vi "Load Flattened Image from Tiff.vi"(0 "path to TIFF file":path=path "/HD1/Users/herbertlooser/Desktop/LadungssprŸher.tif", 1 "error in (no error)":errorcluster) -> (5 "image data":T1, 7 "error out":errorcluster)   [LabVIEW 2012, in "TIFF File Reader.lvlib"]
uses:
  TIFF File Reader.lvlib
  <vilib>/picture/picture.llb/imagedata.ctl
  Globals.vi
panel:
  in  "Tab Control":T2(tab)
  out "Grayscale":picture
  out "Gray16/32":sgl[][](array[numeric])
  out "N_Bits":u64
  out "Gray8":u8[][](array[numeric])
  out "GrayWithLUT":picture
  out "Gray8 LUT":u8[][](array[numeric])
  out "RGB":picture
  out "N_RGB_Bits":u64
  out "R16/32":sgl[][](array[numeric])
  out "G16/32":sgl[][](array[numeric])
  out "B16/32":sgl[][](array[numeric])
  out "RGB8":u32[][](array[numeric])
  out "PhotoM":T3(ring)=enum."BlackIsZero"
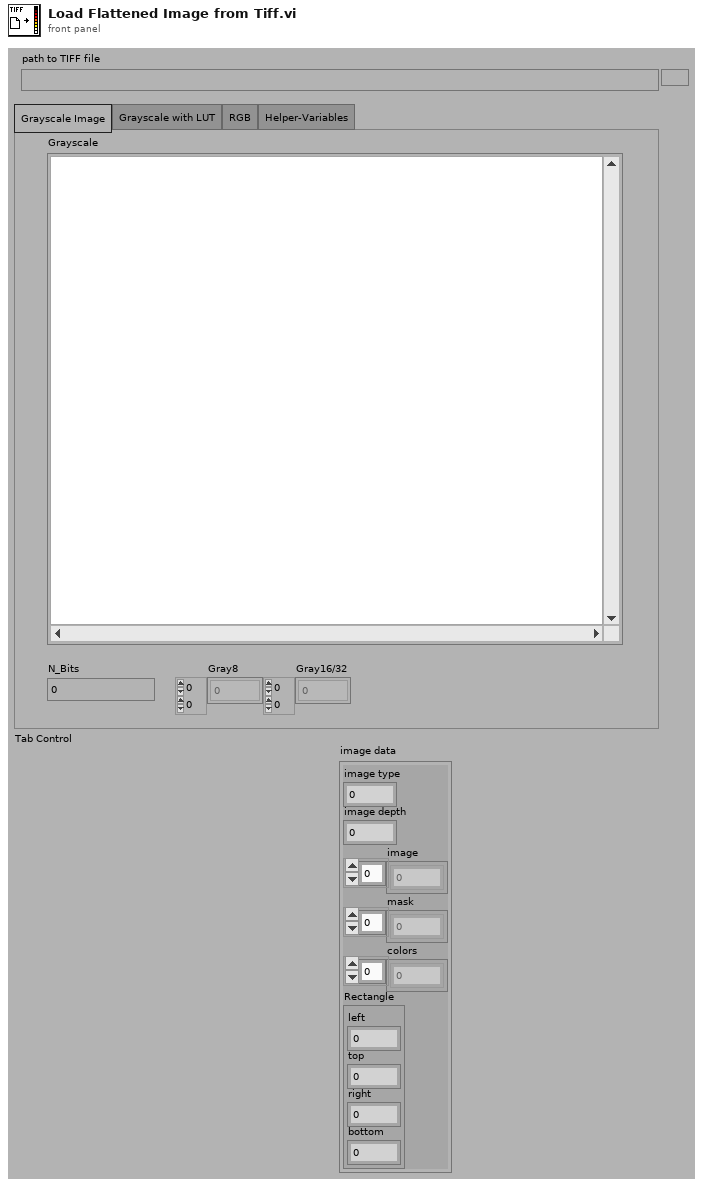
[diagram p1: front panel]
types:
  T1 = typedef "imagedata.ctl" = cluster{"image type":i32, "image depth":i32, "image":u8[], "mask":u8[], "colors":u32[], "Rectangle":cluster{"left":i16, "top":i16, "right":i16, "bottom":i16}}
  T2 = enum32{"Grayscale Image", "Grayscale with LUT", "RGB", "Helper-Variables"}
  T3 = enum16{"WhiteIsZero", "BlackIsZero", "RGB", "RGBPalette", "TranspMask", "CMYK", "YCbCr", "Null", "CIELab"}
  T4 = enum16{"open", "open or create", "create or replace", "create"}
  T5 = enum32{"existing file", "new file", "new or existing file", "existing dir", "new dir", "new or existing dir", "existing file (use LLBs)", "new file (use LLBs)", "new or existing file (use LLBs)", "new or existing file or directory (use LLBs)", "existing dir (use LLBs)", "new dir (use LLBs)", "new or existing dir (use LLBs)", "existing file or dir", "new file or dir", "new or existing file or dir", "existing file or dir (use LLBs)", "new file or dir (use LLBs)"}
  T6 = typedef "TIFF File Reader.lvlib/IFD Entry.ctl" = cluster{"Tag":u16, "Type":T7, "Count":u32, "Val/Offs":u32, "Is Val/Offs(T)":bool}
  T7 = typedef "TIFF File Reader.lvlib/FieldTypes.ctl" = enum16{"NULL", "U8", "ASCII7", "U16", "U32", "RATIONAL", "SByte(I8)", "Undef(8Bit)", "I16", "I32", "SRat(4B:4B)", "SGL(4Byte)", "DBL(8Byte)"}
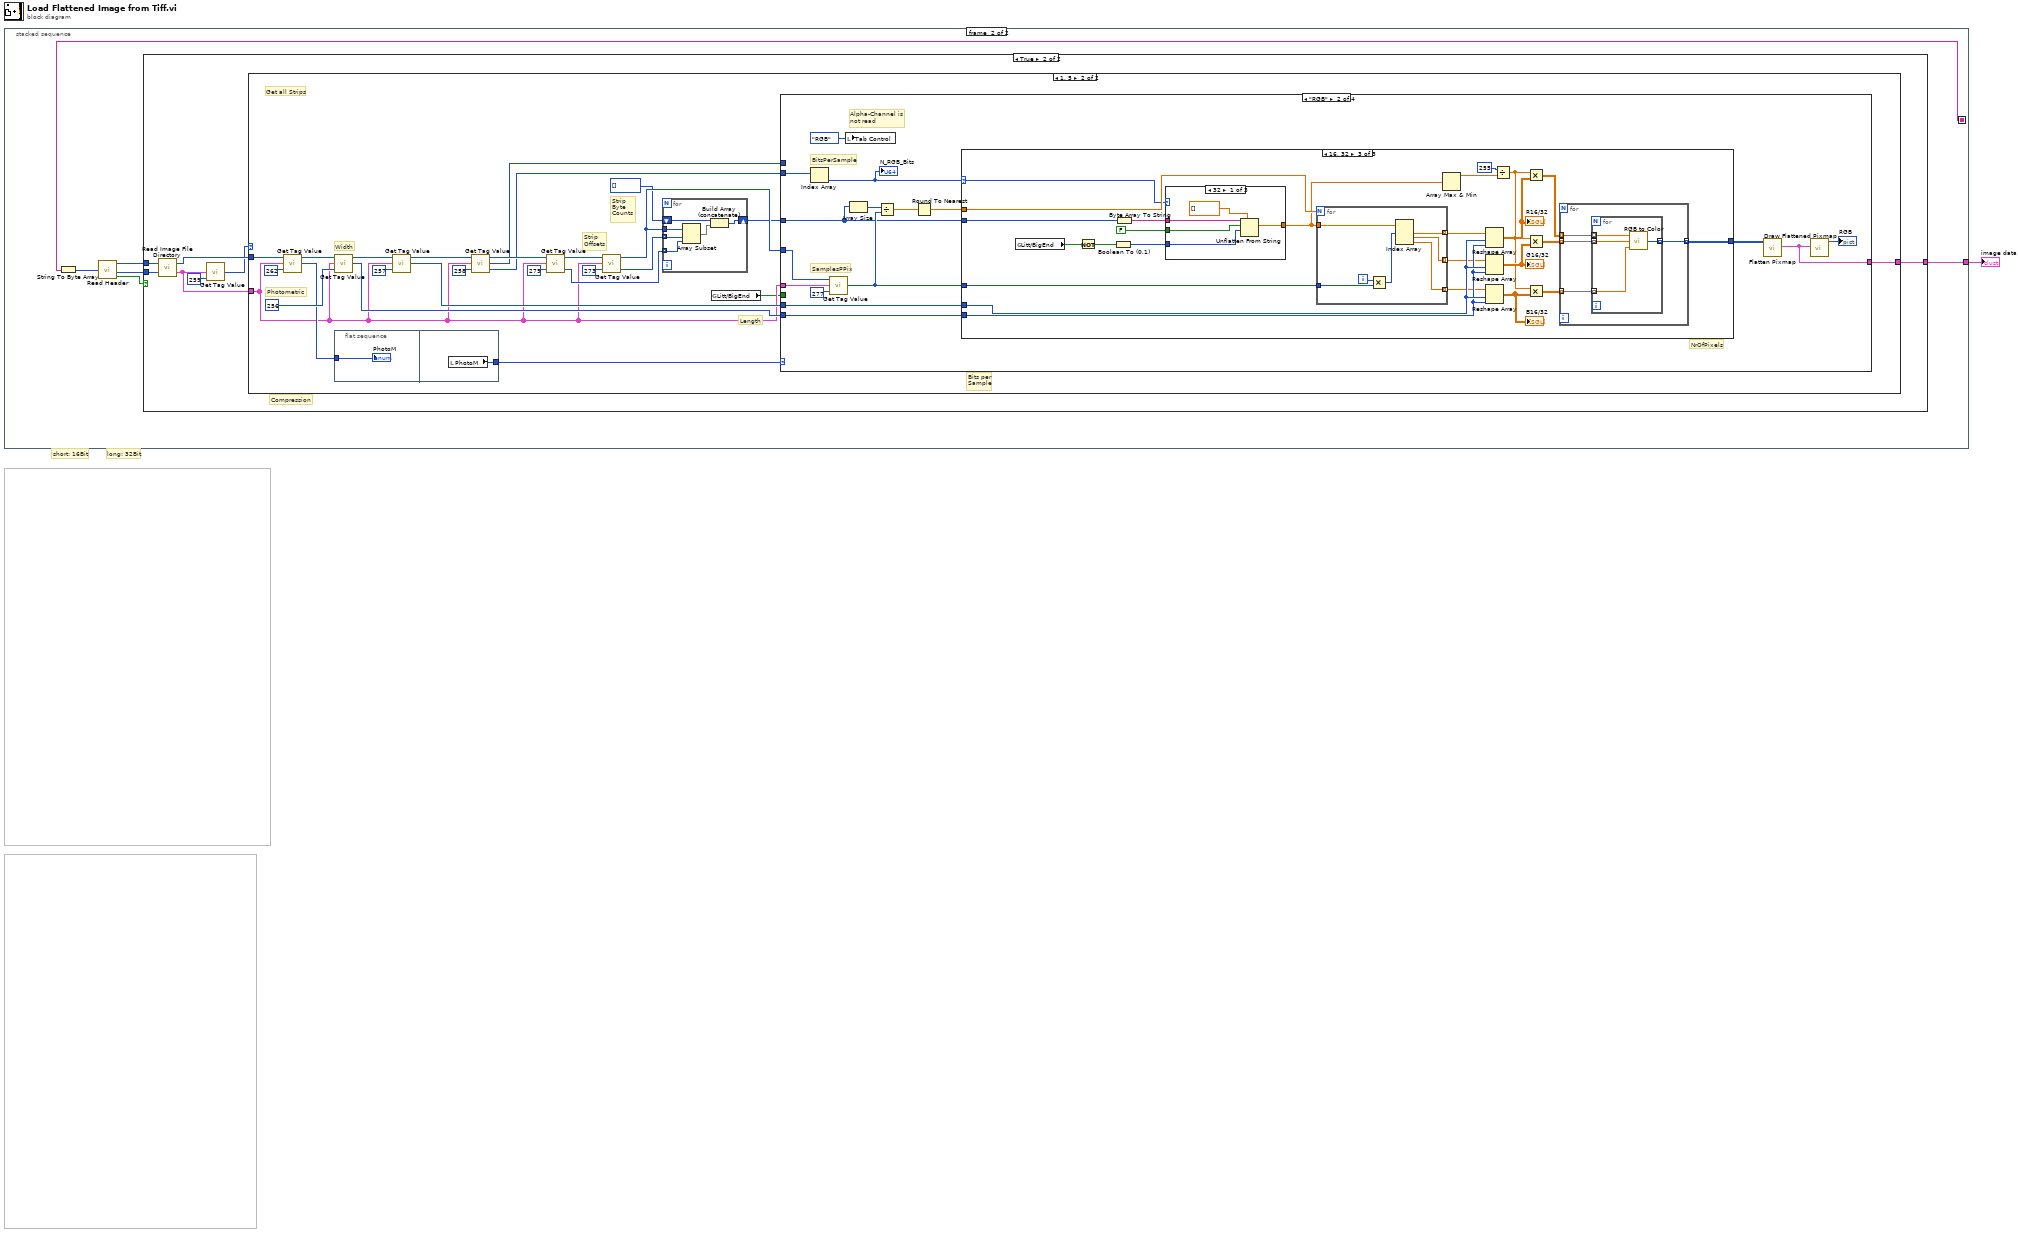
[diagram p0: block diagram]
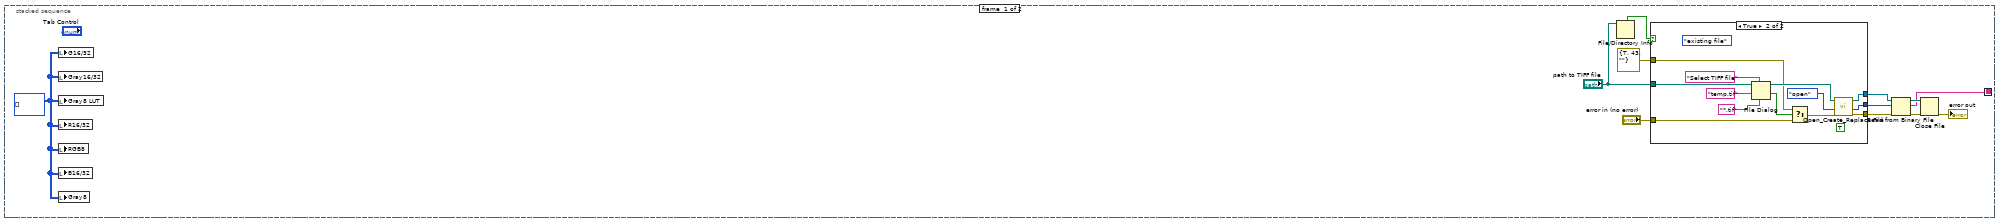
[diagram p2: hidden frame]
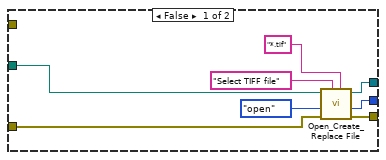
[diagram p3: hidden frame]
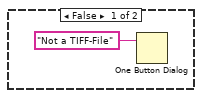
[diagram p4: hidden frame]
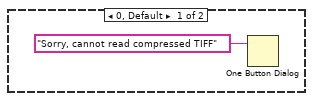
[diagram p5: hidden frame]
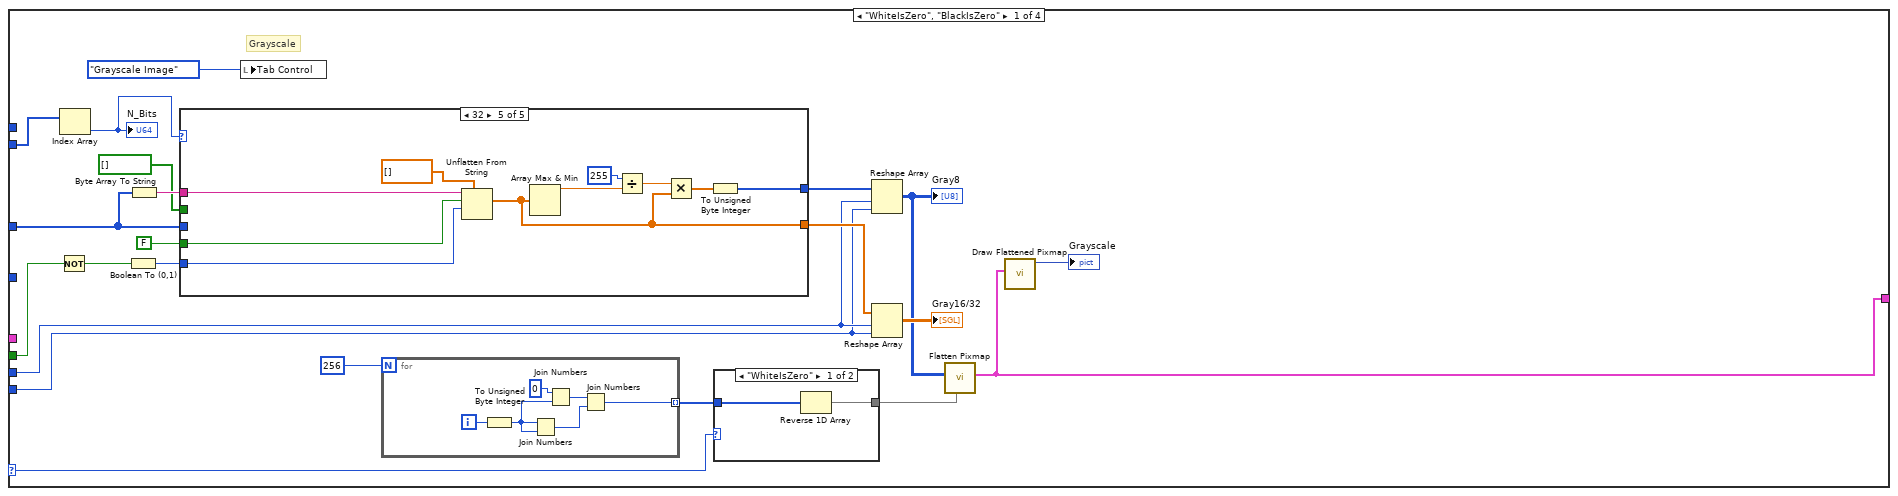
[diagram p6: hidden frame]
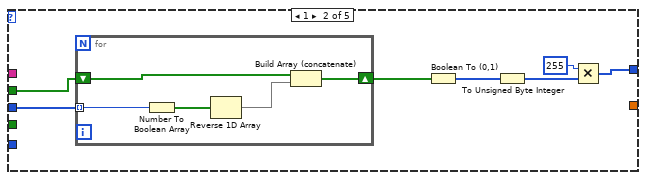
[diagram p9: hidden frame]
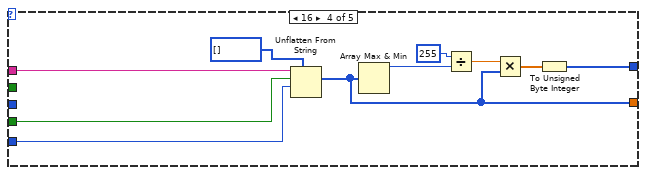
[diagram p11: hidden frame]
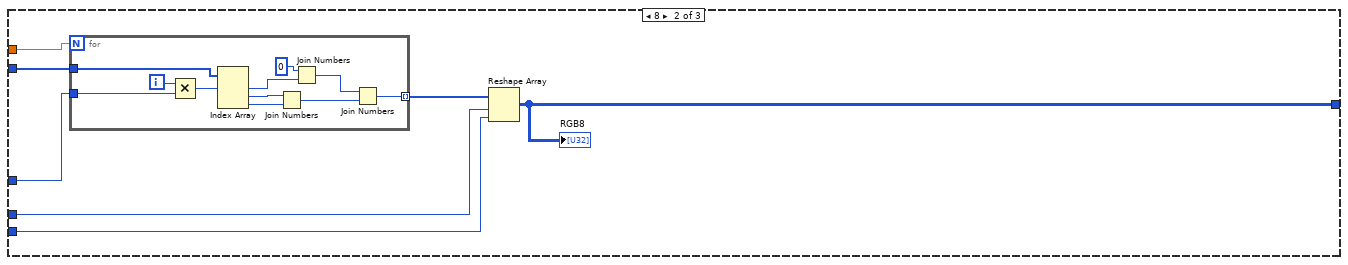
[diagram p13: hidden frame]
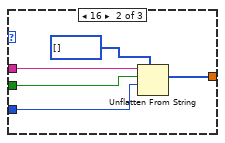
[diagram p14: hidden frame]
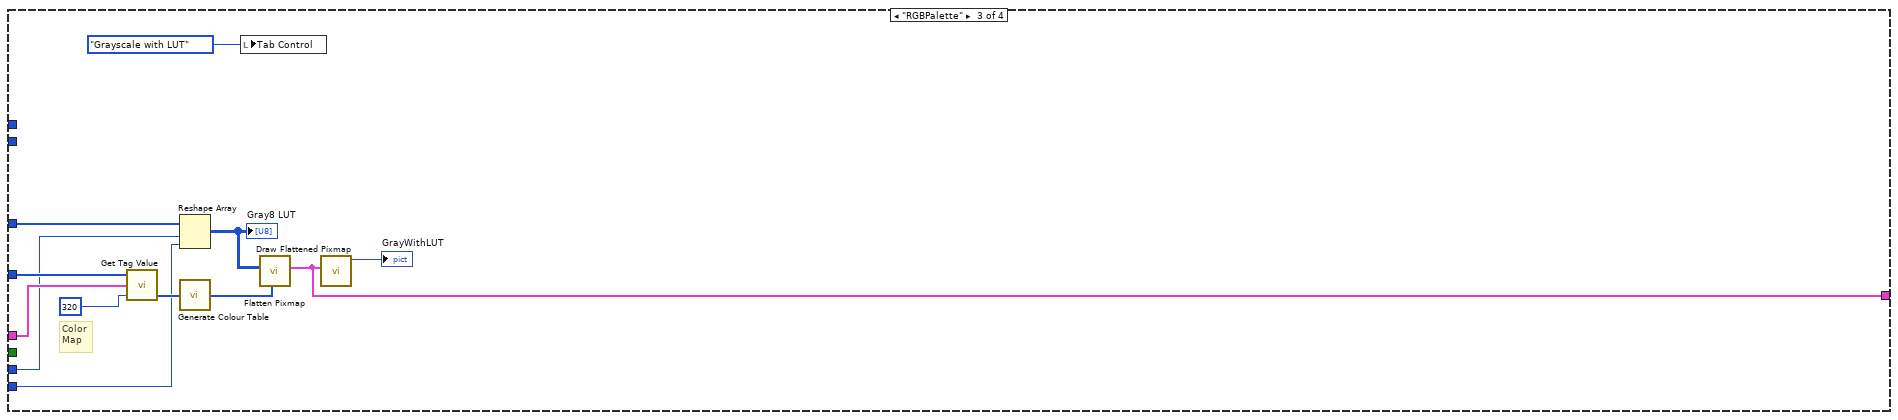
[diagram p16: hidden frame]
diagram:
  # "long: 32Bit"
  # "short: 16Bit"
  n1 = stacked-sequence {
    seq-local: [w3 _] -> [_ w39]
    tunnel: [_ w35] -> w1
    frame #0 {
      w2 = u32[][] [] ("RGB8")
      n2 = local write "G16/32"(w2) -> ()
      n3 = local write "Gray16/32"(w2) -> ()
      n4 = local write "Gray8 LUT"(w2) -> ()
      n5 = local write "R16/32"(w2) -> ()
      n6 = local write "RGB8"(w2) -> ()
      n7 = local write "B16/32"(w2) -> ()
      n8 = local write "Gray8"(w2) -> ()
      n9 = File/Directory Info(path="path to TIFF file") -> (directory=w7:bool)  [unwired: 1 in, 6 out]
      n10 = case shown="True" w7 {
        tunnel: [w18 w27] -> w13
        tunnel: [w17 w29] -> w12
        tunnel: [w16 w28] -> w9
        tunnel: "error in (no error)" -> [w15 w25]
        tunnel: "path to TIFF file" -> [w14 w22]
        tunnel: errorcluster {"status"=TRUE, "code"=43, "source"=""} ("error in (no error)") -> [_ w23]
        frame False {
          n11 = call <vilib>:"Open_Create_Replace File.vi"("pattern"="*.tif", "prompt"="Select TIFF file", "error in (no error)"=w15, "function (open:0)"=T4."open", "file path"=w14) -> ("error out"=w16:errorcluster, "file size (bytes)"=w18:i32, "refnum"=w17:refnum<file>)  [unwired: 2 in, 2 out]
        }
        frame True {
          (unwired) T5."existing file" ("select mode (2)")
          (unwired) TRUE ("advisory dialog? (display:T)")
          n12 = File Dialog(6:"*.tif" ("pattern"), 7:"Select TIFF file" ("prompt"), 9:"temp.tif" ("default name"), 11:w22) -> (1:w26:bool, 3:w31:path)  [unwired: 1 in, 4 out]
          n13 = Select(t=w23, s=w26, f=w25) -> (s? t:f=w24:errorcluster)
          n14 = call <vilib>:"Open_Create_Replace File.vi"("error in (no error)"=w24, "function (open:0)"=T4."open", "file path"=w31) -> ("error out"=w28:errorcluster, "file size (bytes)"=w27:i32, "refnum"=w29:refnum<file>)  [unwired: 3 in, 3 out]
        }
      }
      n15 = Read from Binary File(8:w9, 10:w13, 11:w12) -> (0:w10:errorcluster, 2:w3:string, 3:w11:refnum<file>)  [unwired: 4 out]
      n16 = Close File(refnum=w11, error in=w10) -> (error out=→"error out":errorcluster)  [unwired: 1 out]
    }
    frame #1 {
      n17 = String To Byte Array(string=w39) -> (unsigned byte array=w40:u8[])
      n18 = call "Read Header.vi"("Image Data in"=w40) -> ("Image Data out"=w38:u8[], "ImFileDirectOffs"=w37:u32, "isTIFF"=w36:bool)  [unwired: 1 out]
      n19 = case shown="True" w36 {
        tunnel: w38 -> [_ w48]
        tunnel: w37 -> [_ w47]
        tunnel: [_ w42] -> w35
        frame False {
          n20 = One Button Dialog(message="Not a TIFF-File") -> ()  [unwired: 2 out]
        }
        frame True {
          # "Compression"
          n21 = call "Read Image File Directory.vi"("Im_File_Dir Offs"=w47, "Image Data in"=w48) -> ("Directory"=w43:T6[], "Image Data out"=w46:u8[])
          n22 = call "Get Tag Value.vi"("Tag Code"=u16 259, "DirEntries"=w43) -> ("Single Value"=w44:u32)  [unwired: 1 in, 2 out]
          n23 = case shown="1, 5" w44 {
            tunnel: w46 -> [_ w70]
            tunnel: w43 -> [_ w52]
            tunnel: [_ w50] -> w42
            frame 0, Default {
              n24 = One Button Dialog(message="Sorry, cannot read compressed TIFF") -> ()  [unwired: 2 out]
            }
            frame 1, 5 {
              # "Get all Strips"
              # "Strip\nOffsets"
              # "Strip\nByte\nCounts"
              # "Bits per\nSample"
              # "Photometric"
              # "Length"
              # "Width"
              n25 = call "Get Tag Value.vi"("Tag Code"=u16 262, "DirEntries"=w52, "Image Data in"=w70) -> ("Single Value"=w59:u32, "Image Data out"=w69:u8[])  [unwired: 1 out]
              n26 = call "Get Tag Value.vi"("Tag Code"=u16 256, "DirEntries"=w52, "Image Data in"=w69) -> ("Single Value"=w71:u32, "Image Data out"=w75:u8[])  [unwired: 1 out]
              n27 = flat-sequence {
                tunnel: w59 -> [w82]
                tunnel: [w83] -> w58
                frame #0 {
                  "PhotoM" <- w82
                }
                frame #1 {
                  n28 = local read "PhotoM"() -> (w83:T3)
                }
              }
              n29 = call "Get Tag Value.vi"("Tag Code"=u16 257, "DirEntries"=w52, "Image Data in"=w75) -> ("Single Value"=w72:u32, "Image Data out"=w66:u8[])  [unwired: 1 out]
              n30 = call "Get Tag Value.vi"("Tag Code"=u16 258, "DirEntries"=w52, "Image Data in"=w66) -> ("Multiple Values"=w60:u64[], "Single Value"=w61:u32, "Image Data out"=w65:u8[])
              n31 = call "Get Tag Value.vi"("Tag Code"=u16 279, "DirEntries"=w52, "Image Data in"=w65) -> ("Multiple Values"=w55:u64[], "Image Data out"=w64:u8[])  [unwired: 1 out]
              n32 = call "Get Tag Value.vi"("Tag Code"=u16 273, "DirEntries"=w52, "Image Data in"=w64) -> ("Multiple Values"=w56:u64[], "Image Data out"=w57:u8[])  [unwired: 1 out]
              n33 = for {
                tunnel: w57 -> [w81]
                tunnel: w56 -> [w80] mode=indexing
                tunnel: w55 -> [w79] mode=indexing
                shift-right: [w78] -> w53
                shift-left: u8[] [] -> [w76]
                n34 = Array Subset(array=w81, index=w80, length=w79) -> (w77:u8[])
                n35 = Build Array (concatenate)(w76, w77) -> (w78:u8[])
              }
              n36 = global read "Globals.vi" "Litt/BigEnd"() -> (w51:bool)
              n37 = case shown="\"RGB\"" w58 {
                selector: w58 -> [w94 _ _ _]
                tunnel: w72 -> [w93 w163 w239 _]
                tunnel: w57 -> [_ w161 w240 _]
                tunnel: w71 -> [w92 w162 w238 _]
                tunnel: w52 -> [_ w160 w243 _]
                tunnel: w61 -> [_ _ _ _]
                tunnel: w60 -> [w101 w158 _ _]
                tunnel: w53 -> [w100 w150 w237 _]
                tunnel: w51 -> [w86 _ _ _]
                tunnel: [w84 w148 w232 _] -> w50
                frame "WhiteIsZero", "BlackIsZero" {
                  # "Grayscale"
                  n38 = Not(x=w86) -> (.not. x?=w102:bool)
                  n39 = Index Array(array=w101) -> (element=w91:u64)  [unwired: 1 in]
                  "N_Bits" <- w91
                  n40 = Boolean To (0,1)(Boolean=w102) -> (0, 1=w103:i16)
                  n41 = Byte Array To String(unsigned byte array=w100) -> (string=w105:string)
                  n42 = case shown="32" w91 {
                    tunnel: w105 -> [_ _ _ w137 w146]
                    tunnel: [_ _ w127 w128 w139] -> w98
                    tunnel: FALSE ("data includes array or string size? (T)") -> [_ _ _ w136 w145]
                    tunnel: w103 -> [_ _ _ w135 w144]
                    tunnel: w100 -> [_ w121 w127 _ _]
                    tunnel: [_ w116 w127 w129 w140] -> w99
                    tunnel: bool[] [] -> [_ w115 _ _ _]
                    frame 0, 4, Default {
                      # "not\nsupported"
                    }
                    frame 1 {
                      n43 = for {
                        tunnel: w121 -> [w126] mode=indexing
                        shift-right: [w125] -> w120
                        shift-left: w115 -> [w124]
                        n44 = Number To Boolean Array(number=w126) -> (Boolean array=w123:bool[])
                        n45 = Reverse 1D Array(array=w123) -> (reversed array=w122:bool[])
                        n46 = Build Array (concatenate)(w124, w122) -> (w125:bool[])
                      }
                      n47 = Boolean To (0,1)(Boolean=w120) -> (0, 1=w119:i16[])
                      n48 = To Unsigned Byte Integer(number=w119) -> (unsigned 8bit integer=w118:u8[])
                      n49 = Multiply(x=u8 255, y=w118) -> (x*y=w116:u8[])
                    }
                    frame 8 {
                    }
                    frame 16 {
                      n50 = Unflatten From String(type=u16[] [], binary string=w137, data includes array or string size? (T)=w136, byte order (0:big-endian, network order)=w135) -> (value=w128:u16[])  [unwired: 1 in, 2 out]
                      n51 = Array Max & Min(array=w128) -> (max value=w133:u16)  [unwired: 3 out]
                      n52 = Divide(x=255 ("Numeric"), y=w133) -> (x/y=w132:dbl)
                      n53 = Multiply(x=w132, y=w128) -> (x*y=w130:dbl[])
                      n54 = To Unsigned Byte Integer(number=w130) -> (unsigned 8bit integer=w129:u8[])
                    }
                    frame 32 {
                      n55 = Unflatten From String(type=sgl[] [], binary string=w146, data includes array or string size? (T)=w145, byte order (0:big-endian, network order)=w144) -> (value=w139:sgl[])  [unwired: 1 in, 2 out]
                      n56 = Array Max & Min(array=w139) -> (max value=w143:sgl)  [unwired: 3 out]
                      n57 = Divide(x=255 ("Numeric"), y=w143) -> (x/y=w142:sgl)
                      n58 = Multiply(x=w142, y=w139) -> (x*y=w141:sgl[])
                      n59 = To Unsigned Byte Integer(number=w141) -> (unsigned 8bit integer=w140:u8[])
                    }
                  }
                  n60 = local write "Tab Control"(T2."Grayscale Image" ("Tab Control")) -> ()
                  n61 = for {
                    N: 256 -> [_]
                    tunnel: [w109] -> w96 mode=indexing
                    i -> [w114]
                    n62 = To Unsigned Byte Integer(number=w114) -> (unsigned 8bit integer=w112:u8)
                    n63 = Join Numbers(hi=w112, lo=w112) -> ((hi.lo)=w111:u16)
                    n64 = Join Numbers(hi=u8 0, lo=w112) -> ((hi.lo)=w110:u16)
                    n65 = Join Numbers(hi=w110, lo=w111) -> ((hi.lo)=w109:u32)
                  }
                  n66 = case shown="\"WhiteIsZero\"" w94 {
                    tunnel: w96 -> [w107 w108]
                    tunnel: [w106 w108] -> w95
                    frame "WhiteIsZero" {
                      n67 = Reverse 1D Array(array=w107) -> (reversed array=w106:u32[])
                    }
                    frame "BlackIsZero", Default {
                    }
                  }
                  n68 = Reshape Array(w99, w93, w92) -> (w87:u8[][])
                  "Gray8" <- w87
                  n69 = Reshape Array(w98, w93, w92) -> (→"Gray16/32":sgl[][])
                  n70 = call <vilib>:"Flatten Pixmap.vi"("colors"=w95, "8-bit pixmap"=w87) -> ("image data"=w84:T1)  [unwired: 4 in, 5 out]
                  n71 = call <vilib>:"Draw Flattened Pixmap.vi"("image data"=w84) -> ("new picture"=→"Grayscale":picture)  [unwired: 1 in, 7 out]
                }
                frame "RGB" {
                  # "BitsPerSample"
                  # "NrOfPixels"
                  # "Alpha-Channel is\nnot read"
                  # "SamplesPPix"
                  n72 = Index Array(array=w158) -> (element=w153:u64)  [unwired: 1 in]
                  "N_RGB_Bits" <- w153
                  n73 = call "Get Tag Value.vi"("Tag Code"=u16 277, "DirEntries"=w160, "Image Data in"=w161) -> ("Single Value"=w155:u32)  [unwired: 2 out]
                  n74 = local write "Tab Control"(T2."RGB" ("Tab Control")) -> ()
                  n75 = Array Size(array=w150) -> (size(s)=w149:i32)
                  n76 = Divide(x=w149, y=w155) -> (x/y=w157:dbl)
                  n77 = Round To Nearest(number=w157) -> (nearest integer value=w156:dbl)
                  n78 = case shown="16, 32" w153 {
                    selector: w153 -> [_ _ w198]
                    tunnel: w163 -> [_ w169 w206]
                    tunnel: w162 -> [_ w168 w205]
                    tunnel: w155 -> [_ w167 w202]
                    tunnel: w150 -> [_ w166 w197]
                    tunnel: w156 -> [_ w165 w203]
                    tunnel: [_ w164 w183] -> w151
                    frame 0, Default {
                    }
                    frame 8 {
                      n79 = for {
                        N: w165 -> [_]
                        tunnel: w166 -> [w181]
                        tunnel: [w174] -> w170 mode=indexing
                        tunnel: w167 -> [w171]
                        i -> [w172]
                        n80 = Multiply(x=w172, y=w171) -> (x*y=w173:u32)
                        n81 = Index Array(array=w181, index #1=w173) -> (element #1=w180:u8, element #2=w179:u8, element #3=w178:u8)  [unwired: 2 in]
                        n82 = Join Numbers(hi=w179, lo=w178) -> ((hi.lo)=w176:u16)
                        n83 = Join Numbers(hi=u8 0, lo=w180) -> ((hi.lo)=w175:u16)
                        n84 = Join Numbers(hi=w175, lo=w176) -> ((hi.lo)=w174:u32)
                      }
                      n85 = Reshape Array(w170, w169, w168) -> (w164:u32[][])
                      "RGB8" <- w164
                    }
                    frame 16, 32 {
                      n86 = global read "Globals.vi" "Litt/BigEnd"() -> (w182:bool)
                      n87 = Not(x=w182) -> (.not. x?=w199:bool)
                      n88 = Boolean To (0,1)(Boolean=w199) -> (0, 1=w200:i16)
                      n89 = Byte Array To String(unsigned byte array=w197) -> (string=w204:string)
                      n90 = case shown="32" w198 {
                        tunnel: w204 -> [w219 w224 _]
                        tunnel: [w215 w223 _] -> w193
                        tunnel: FALSE ("data includes array or string size? (T)") -> [w218 w222 _]
                        tunnel: w200 -> [w217 w221 _]
                        frame 32 {
                          n91 = Unflatten From String(type=sgl[] [], binary string=w219, data includes array or string size? (T)=w218, byte order (0:big-endian, network order)=w217) -> (value=w215:sgl[])  [unwired: 1 in, 2 out]
                        }
                        frame 16 {
                          n92 = Unflatten From String(type=u16[] [], binary string=w224, data includes array or string size? (T)=w222, byte order (0:big-endian, network order)=w221) -> (value=w223:u16[])  [unwired: 1 in, 2 out]
                        }
                        frame 0, Default {
                        }
                      }
                      n93 = for {
                        N: w203 -> [_]
                        tunnel: w193 -> [w231]
                        tunnel: [w230] -> w192 mode=indexing
                        tunnel: [w229] -> w196 mode=indexing
                        tunnel: [w228] -> w195 mode=indexing
                        tunnel: w202 -> [w225]
                        i -> [w226]
                        n94 = Multiply(x=w226, y=w225) -> (x*y=w227:u32)
                        n95 = Index Array(array=w231, index #1=w227) -> (element #1=w230:sgl, element #2=w229:sgl, element #3=w228:sgl)  [unwired: 2 in]
                      }
                      n96 = Array Max & Min(array=w193) -> (max value=w191:sgl)  [unwired: 3 out]
                      n97 = Reshape Array(w192, w206, w205) -> (w190:sgl[][])
                      "R16/32" <- w190
                      n98 = Reshape Array(w196, w206, w205) -> (w189:sgl[][])
                      "G16/32" <- w189
                      n99 = Reshape Array(w195, w206, w205) -> (w188:sgl[][])
                      "B16/32" <- w188
                      n100 = Divide(x=255, y=w191) -> (x/y=w187:sgl)
                      n101 = Multiply(x=w187, y=w190) -> (x*y=w186:sgl[][])
                      n102 = Multiply(x=w187, y=w189) -> (x*y=w185:sgl[][])
                      n103 = Multiply(x=w187, y=w188) -> (x*y=w184:sgl[][])
                      n104 = for {
                        tunnel: w186 -> [w210] mode=indexing
                        tunnel: w185 -> [w209] mode=indexing
                        tunnel: w184 -> [w208] mode=indexing
                        tunnel: [w207] -> w183 mode=indexing
                        n105 = for {
                          tunnel: w210 -> [w214] mode=indexing
                          tunnel: w209 -> [w213] mode=indexing
                          tunnel: w208 -> [w212] mode=indexing
                          tunnel: [w211] -> w207 mode=indexing
                          n106 = call <vilib>:"RGB to Color.vi"("B"=w212, "G"=w213, "R"=w214) -> ("Color"=w211:u32)
                        }
                      }
                    }
                  }
                  n107 = call <vilib>:"Flatten Pixmap.vi"("24-bit pixmap"=w151) -> ("image data"=w148:T1)  [unwired: 5 in, 5 out]
                  n108 = call <vilib>:"Draw Flattened Pixmap.vi"("image data"=w148) -> ("new picture"=→"RGB":picture)  [unwired: 1 in, 7 out]
                }
                frame "RGBPalette" {
                  # "Color\nMap"
                  n109 = call "Get Tag Value.vi"("Tag Code"=u16 320, "DirEntries"=w243, "Image Data in"=w240) -> ("Multiple Values"=w242:u64[])  [unwired: 2 out]
                  n110 = Reshape Array(w237, w239, w238) -> (w233:u8[][])
                  "Gray8 LUT" <- w233
                  n111 = call "Generate Colour Table.vi"("Code 320 Values"=w242) -> ("Colour Table"=w236:u32[])
                  n112 = local write "Tab Control"(T2."Grayscale with LUT" ("Tab Control")) -> ()
                  n113 = call <vilib>:"Flatten Pixmap.vi"("colors"=w236, "8-bit pixmap"=w233) -> ("image data"=w232:T1)  [unwired: 4 in, 5 out]
                  n114 = call <vilib>:"Draw Flattened Pixmap.vi"("image data"=w232) -> ("new picture"=→"GrayWithLUT":picture)  [unwired: 1 in, 7 out]
                }
                frame "TranspMask".."CIELab" {
                  # "unsupported"
                }
              }
            }
          }
        }
      }
    }
  }
  "image data" <- w1
